vi "Execute.vi"(6 "Index [-1]":i32=-1, 7 "Composite Object":refnum<class "CConfig Object.lvclass">, 8 "error in (no error)":errorcluster, 9 "Results":string[][](array[string]), 11 "Config Query in":refnum<class "Loop Query.lvclass">) -> (0 "error out":errorcluster, 1 "Results":string[][](array[string]), 2 "Result":bool, 3 "Config Query out":refnum<class "Loop Query.lvclass">, 4 "Index":i32, 5 "Composite Object":refnum<class "CConfig Object.lvclass">)   [LabVIEW 2013, in "Loop Query.lvclass"]
doc: "Copyright 2018, Carya Automatisering, Wiebe Walstra."
uses:
  Loop Query.lvclass
  CConfig Object.lvclass
  Loop Query.lvclass/Loop Query.ctl
  CConfig Query.lvclass
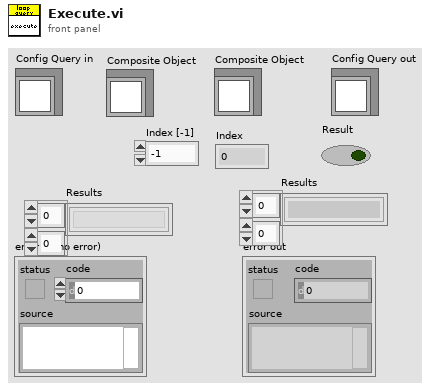
[diagram p1: front panel]
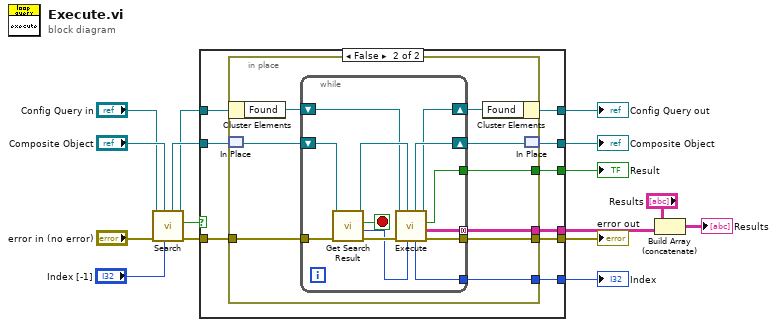
[diagram p0: block diagram]
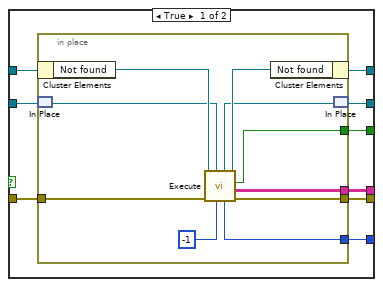
[diagram p2: hidden frame]
diagram:
  n1 = call-dynamic "Search.vi"("Index in"="Index [-1]", "Composite Object"="Composite Object", "error in (no error)"="error in (no error)", "Find Query in"="Config Query in") -> ("error out"=w10:errorcluster, "empty?"=w4:bool, "Find Query out"=w1:refnum<class "Loop Query.lvclass">, "Composite Object"=w11:refnum<class "CConfig Object.lvclass">)  [unwired: 4 in]
  n2 = case shown="False" w4 {
    tunnel: [w22 w41] -> w3
    tunnel: w1 -> [w23 w42]
    tunnel: w10 -> [w25 w44]
    tunnel: [w24 w43] -> w8
    tunnel: w11 -> [w18 w37]
    tunnel: [w17 w36] -> w6
    tunnel: [w21 w40] -> w5
    tunnel: [w20 w39] -> w7
    tunnel: [w19 w38] -> w9
    frame True {
      n3 = in-place {
        in-place-border: w25 -> [w35]
        in-place-border: [w34] -> w24
        in-place-border: [w31] -> w21
        in-place-border: [w30] -> w20
        in-place-border: [w29] -> w19
        n4 = in-place-cluster #1(w23) -> ("Not found"=w33:refnum<class "CConfig Query.lvclass">)
        n5 = in-place-match #2(w18) -> (w27:refnum<class "CConfig Object.lvclass">)
        n6 = call-dynamic "Execute.vi"("Index [-1]"=-1, "Composite Object"=w27, "error in (no error)"=w35, "Config Query in"=w33) -> ("error out"=w34:errorcluster, "Results"=w29:string[][], "Result"=w31:bool, "Config Query out"=w32:refnum<class "CConfig Query.lvclass">, "Index"=w30:i32, "Composite Object"=w26:refnum<class "CConfig Object.lvclass">)  [unwired: 2 in]
        n7 = in-place-cluster #1("Not found"=w32) -> (w22:refnum<class "Loop Query.lvclass">)
        n8 = in-place-match #2(w26) -> (w17:refnum<class "CConfig Object.lvclass">)
      }
    }
    frame False {
      n9 = in-place {
        in-place-border: w44 -> [w53]
        in-place-border: [w52] -> w43
        in-place-border: [w50] -> w40
        in-place-border: [w49] -> w39
        in-place-border: [w48] -> w38
        n10 = in-place-cluster #3(w42) -> ("Found"=w47:refnum<class "CConfig Query.lvclass">)
        n11 = in-place-match #4(w37) -> (w46:refnum<class "CConfig Object.lvclass">)
        n12 = while {
          tunnel: w53 -> [w66]
          tunnel: [w65] -> w52
          tunnel: [w63] -> w50
          tunnel: [w62] -> w49
          tunnel: [w61] -> w48 mode=concatenating
          shift-right: [w64] -> w45
          shift-left: w46 -> [w59]
          shift-right: [w55] -> w51
          shift-left: w47 -> [w56]
          stop <- w57 stop-if-true
          n13 = call-dynamic "Get Search Result.vi"("error in (no error)"=w66, "Composite Object in"=w59) -> ("error out"=w60:errorcluster, "deleted portion"=w54:i32, "empty?"=w57:bool, "Composite Object out"=w58:refnum<class "CConfig Object.lvclass">)  [unwired: 6 in]
          n14 = call-dynamic "Execute.vi"("Index [-1]"=w54, "Composite Object"=w58, "error in (no error)"=w60, "Config Query in"=w56) -> ("error out"=w65:errorcluster, "Results"=w61:string[][], "Result"=w63:bool, "Config Query out"=w55:refnum<class "CConfig Query.lvclass">, "Index"=w62:i32, "Composite Object"=w64:refnum<class "CConfig Object.lvclass">)  [unwired: 2 in]
        }
        n15 = in-place-cluster #3("Found"=w51) -> (w41:refnum<class "Loop Query.lvclass">)
        n16 = in-place-match #4(w45) -> (w36:refnum<class "CConfig Object.lvclass">)
      }
    }
  }
  "error out" <- w8
  "Config Query out" <- w3
  "Composite Object" <- w6
  "Result" <- w5
  "Index" <- w7
  n17 = Build Array (concatenate)("Results", w9) -> (→"Results":string[][])
